vi "NI_FPGA_PPG.publish cmd data.vi"(0 "i ref in":refnum<vi>, 2 "cmd_data_string":string, 3 "ms timeout (10000)":i32=10000, 5 "error in (no error)":errorcluster) -> (14 "i ref out":refnum<vi>, 17 "timed out":bool, 19 "error out":errorcluster)   [LabVIEW 2014, in "NI_FPGA_PPG.lvlib"]
doc: "Publishes a string with the last (pattern-)command received from the host\n\nLicense Agreement for this software:\n\nCopyright (C) 2009\nFalk Ziegler\nInstitut für Physik\nErnst-Moritz-Arndt Universität\nFelix-Hausdorff-Str. 6\n17487 Greifswald\n\nContact: Falk Ziegler, ziegler@physik.uni-greifswald.de\n\nThis program is free software: you can redistribute it and/or modify it under the terms of the GNU General Public License as published by the Free Software Foundation, either version 3 of the License, or (at your option) any later version.\n\nThis program is distributed in the hope that it will be useful, but WITHOUT ANY WARRANTY; without even the implied warranty of MERCHANTABILITY or FITNESS FOR A PARTICULAR PURPOSE. See the GNU General Public License for more details.\n\nYou should have received a copy of the GNU General Public License along with this program. If not, see <http://www.gnu.org/licenses/>.\n\nFor all questions and ideas contact: ziegler@physik.uni-greifswald.de or d.beck@gsi.de\nLast update: 01-Sep-2009"
uses:
  NI_FPGA_PPG.lvlib
  CSlibraries-extern/DimLVEvent/LVDimInterface/LVDimInterface.lvlib
  CSCore/CSSystem/CSSystemLib/CSSystemLib.lvlib
  CSlibraries/UtilityLib/UtilityLib.lvlib
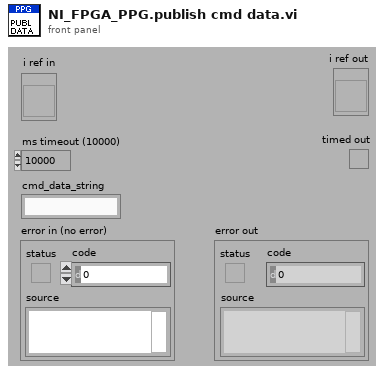
[diagram p1: front panel]
types:
  T1 = typedef "NI_FPGA_PPG.lvlib/NI_FPGA_PPG.i attribute.ctl" = cluster{"dim_service_id":cluster{"dim_actual_device_status":i32, "dim_event_data":i32, "dim_cmd_data":i32, "dim_cmd_data _description":i32, "dim_channel_description":i32}, "VISA":refnum<visa-resource-name>, "actual_device_status":i32, "event_data_id":i32, "pdc_enabled":bool, "pdc_timestamp":u32, "cmd_data_string":string, "cmd_data_size":i32, "cmd_data_description_string":string, "cmd_data_description_size":i32, "channel_description_string":string, "channel_description_size":i32}
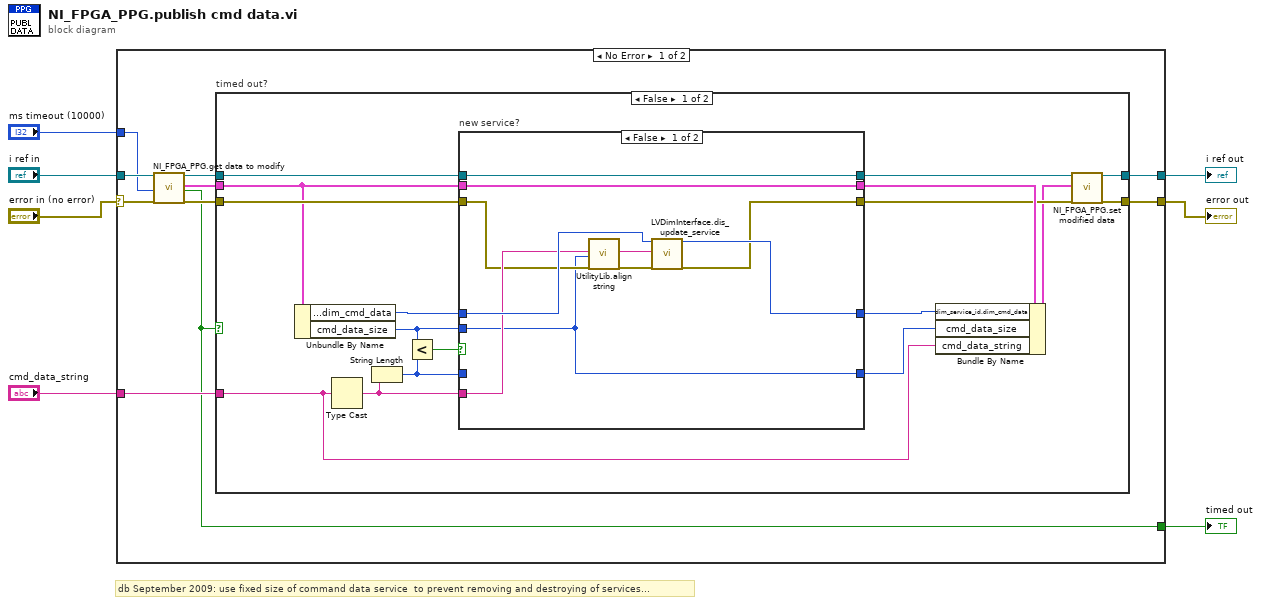
[diagram p0: block diagram]
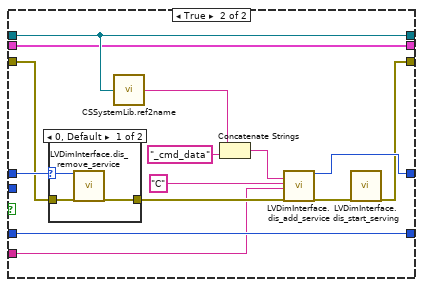
[diagram p2: hidden frame]
diagram:
  # "db September 2009: use fixed size of command data service  to prevent removing and destroying of services..."
  n1 = case shown="No Error" "error in (no error)" {
    selector: "error in (no error)" -> [w14 w64]
    tunnel: "i ref in" -> [w16 w65]
    tunnel: [w17 w65] -> w5
    tunnel: [w9 w64] -> w4
    tunnel: "ms timeout (10000)" -> [w11 _]
    tunnel: "cmd_data_string" -> [w10 _]
    tunnel: [w8 _] -> w1
    frame No Error {
      n2 = call "NI_FPGA_PPG.get data to modify.vi"("i ref in"=w16, "ms timeout (10000)"=w11, "error in (no error)"=w14) -> ("i ref out"=w15:refnum<vi>, "i attribute"=w12:T1, "timed out"=w8:bool, "error out"=w13:errorcluster)  [unwired: 13 in]
      n3 = case "timed out?" shown="False" w8 {
        tunnel: [w29 w63] -> w17
        tunnel: w15 -> [w32 w63]
        tunnel: w13 -> [w31 w62]
        tunnel: w12 -> [w28 _]
        tunnel: w10 -> [w19 _]
        tunnel: [w21 w62] -> w9
        frame False {
          n4 = Unbundle By Name(w28) -> ("dim_service_id.dim_cmd_data"=w33:i32, "cmd_data_size"=w18:i32)
          n5 = Type Cast(x=w19) -> (*(type *) &x=w20:string)  [unwired: 1 in]
          n6 = String Length(string=w20) -> (length=w23:i32)
          n7 = Less?(x=w18, y=w23) -> (x < y?=w34:bool)
          n8 = case "new service?" shown="False" w34 {
            tunnel: w32 -> [w44 w53]
            tunnel: [w44 w53] -> w30
            tunnel: w33 -> [w43 w58]
            tunnel: w31 -> [w36 w54]
            tunnel: w20 -> [w40 w48]
            tunnel: [w42 w52] -> w26
            tunnel: [w41 w51] -> w25
            tunnel: w28 -> [w39 w50]
            tunnel: [w39 w50] -> w27
            tunnel: w23 -> [_ w49]
            tunnel: [w35 w49] -> w22
            tunnel: w18 -> [w35 _]
            frame False {
              n9 = call "UtilityLib.align string.vi"("stringIn"=w40, "stringLength (80)"=w35, "error in (no error)"=w36) -> ("stringOut"=w38:string, "error out"=w37:errorcluster)  [unwired: 15 in]
              n10 = call "LVDimInterface.dis_update_service.vi"("my_serviceID"=w43, "data"=w38, "error in (no error)"=w37) -> ("my_serviceID out"=w42:i32, "error out"=w41:errorcluster)  [unwired: 14 in, 1 out]
            }
            frame True {
              n11 = case shown="0, Default" w58 {
                selector: w58 -> [w61 _]
                tunnel: [w60 _] -> w57
                tunnel: w54 -> [w59 _]
                frame 0, Default {
                  n12 = call "LVDimInterface.dis_remove_service.vi"("my_serviceID"=w61, "error in (no error)"=w59) -> ("error out"=w60:errorcluster)  [unwired: 17 in]
                }
                frame -1 {
                }
              }
              n13 = call "CSSystemLib.ref2name.vi"("obj refnum"=w53) -> ("name"=w46:string)
              n14 = Concatenate Strings(w46, "_cmd_data" ("string")) -> (w45:string)
              n15 = call "LVDimInterface.dis_add_service.vi"("serviceName"=w45, "typeDescriptor"="C", "data"=w48, "error in (no error)"=w57) -> ("my_serviceID"=w52:i32, "error out"=w55:errorcluster)  [unwired: 14 in]
              n16 = call "LVDimInterface.dis_start_serving.vi"("error in (no error)"=w55) -> ("error out"=w51:errorcluster)  [unwired: 17 in, 1 out]
            }
          }
          n17 = Bundle By Name(cluster=w27, "dim_service_id.dim_cmd_data"=w26, "cmd_data_size"=w22, "cmd_data_string"=w19) -> (w24:T1)
          n18 = call "NI_FPGA_PPG.set modified data.vi"("i ref in"=w30, "i attribute"=w24, "error in (no error)"=w25) -> ("i ref out"=w29:refnum<vi>, "error out"=w21:errorcluster)  [unwired: 15 in]
        }
        frame True {
        }
      }
    }
    frame Error {
    }
  }
  "error out" <- w4
  "i ref out" <- w5
  "timed out" <- w1
